vi "Double_Solenoid_Sample.vi"() -> ()   [LabVIEW 2020]
uses:
  <vilib>/Rock Robotics/WPI/Solenoid/WPI_SolenoidChannel.ctl
  <vilib>/Rock Robotics/WPI/Solenoid/WPI_SolenoidValue.ctl
  <vilib>/Rock Robotics/WPI/ThirdParty/JAS_Junk/TrajLib/Timer_New.vi
  <vilib>/Rock Robotics/WPI/Utilities/WPI_GetSetVariantRefNum.vi
  <vilib>/Rock Robotics/WPI/Solenoid/WPI_SolenoidOpenDouble.vi
  <vilib>/Utility/semaphor.llb/Obtain Semaphore Reference.vi
  <vilib>/Rock Robotics/WPI/ThirdParty/JAS_Junk/TrajLib/Timer_Reset.vi
  <vilib>/Rock Robotics/WPI/ThirdParty/JAS_Junk/TrajLib/Timer_Start.vi
  <vilib>/Rock Robotics/WPI/ThirdParty/JAS_Junk/TrajLib/Timer_HasPeriodPassedOnce.vi
  <vilib>/Rock Robotics/WPI/Solenoid/WPI_SolenoidSetEnum.vi
  <vilib>/Rock Robotics/WPI/Solenoid/WPI_SolenoidGetEnum.vi
  <vilib>/Rock Robotics/WPI/ThirdParty/JAS_Junk/TrajLib/Trajectory_Library.lvlib
panel:
  in  "OneShot Time":dbl=0.33 format="%#_13g"
  out "Desired Cmd":T1
  in  "Intake Dmd":bool
  out "Solenoid Value":T1
  in  "Reverse Solenoid Channel":T2=enum."Solenoid 1"
  in  "Forward Solenoid Channel":T2
  in  "Pneumatics Device (def)":u8
  out "Analog  Sensors":cluster{"Analog 0 (V)":dbl, "Analog 1 (V)":dbl}
  out "Pressure Sensors":T3
  out "Compressor Running":bool
  out "Enabled":bool
  out "Solenoid Cmd Chart":cluster{dbl, "mean":dbl}(graph)
  # "Double Solenoid Example"
  # "Set these values before\nexecuting program"
  # "These values can be\nchanged while the \nprogram is running"
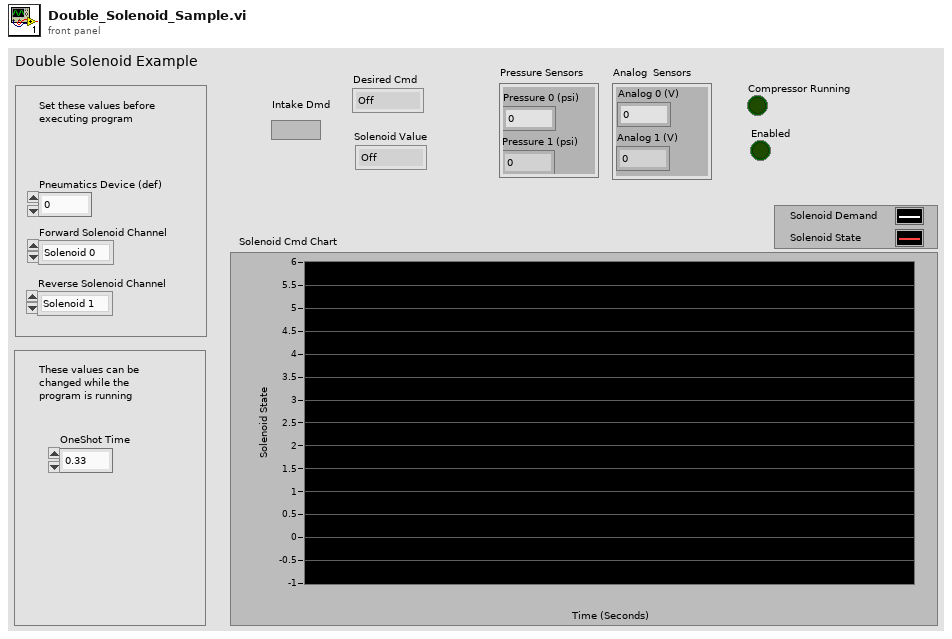
[diagram p1: front panel]
types:
  T1 = typedef "WPI_SolenoidValue.ctl" = enum16{"Off", "On", "Forward", "Reverse"}
  T2 = typedef "WPI_SolenoidChannel.ctl" = enum8{"Solenoid 0", "Solenoid 1", "Solenoid 2", "Solenoid 3", "Solenoid 4", "Solenoid 5", "Solenoid 6", "Solenoid 7", "Solenoid 8", "Solenoid 9", "Solenoid 10", "Solenoid 11", "Solenoid 12", "Solenoid 13", "Solenoid 14", "Solenoid 15", "Invalid"}
  T3 = cluster{"Pressure 0 (psi)":dbl, "Pressure 1 (psi)":dbl}
  T4 = typedef "WPI_CompressorDevRef.ctl" = cluster{"DevStatus":errorcluster, "Pneumatics Control Module":u8}
  T5 = typedef "WPI_SolenoidDevRef.ctl" = cluster{"DevStatus":errorcluster, "Pneumatics Control Module":u8, "Forward Solenoid Channel":T2, "Reverse Solenoid Channel":T2}
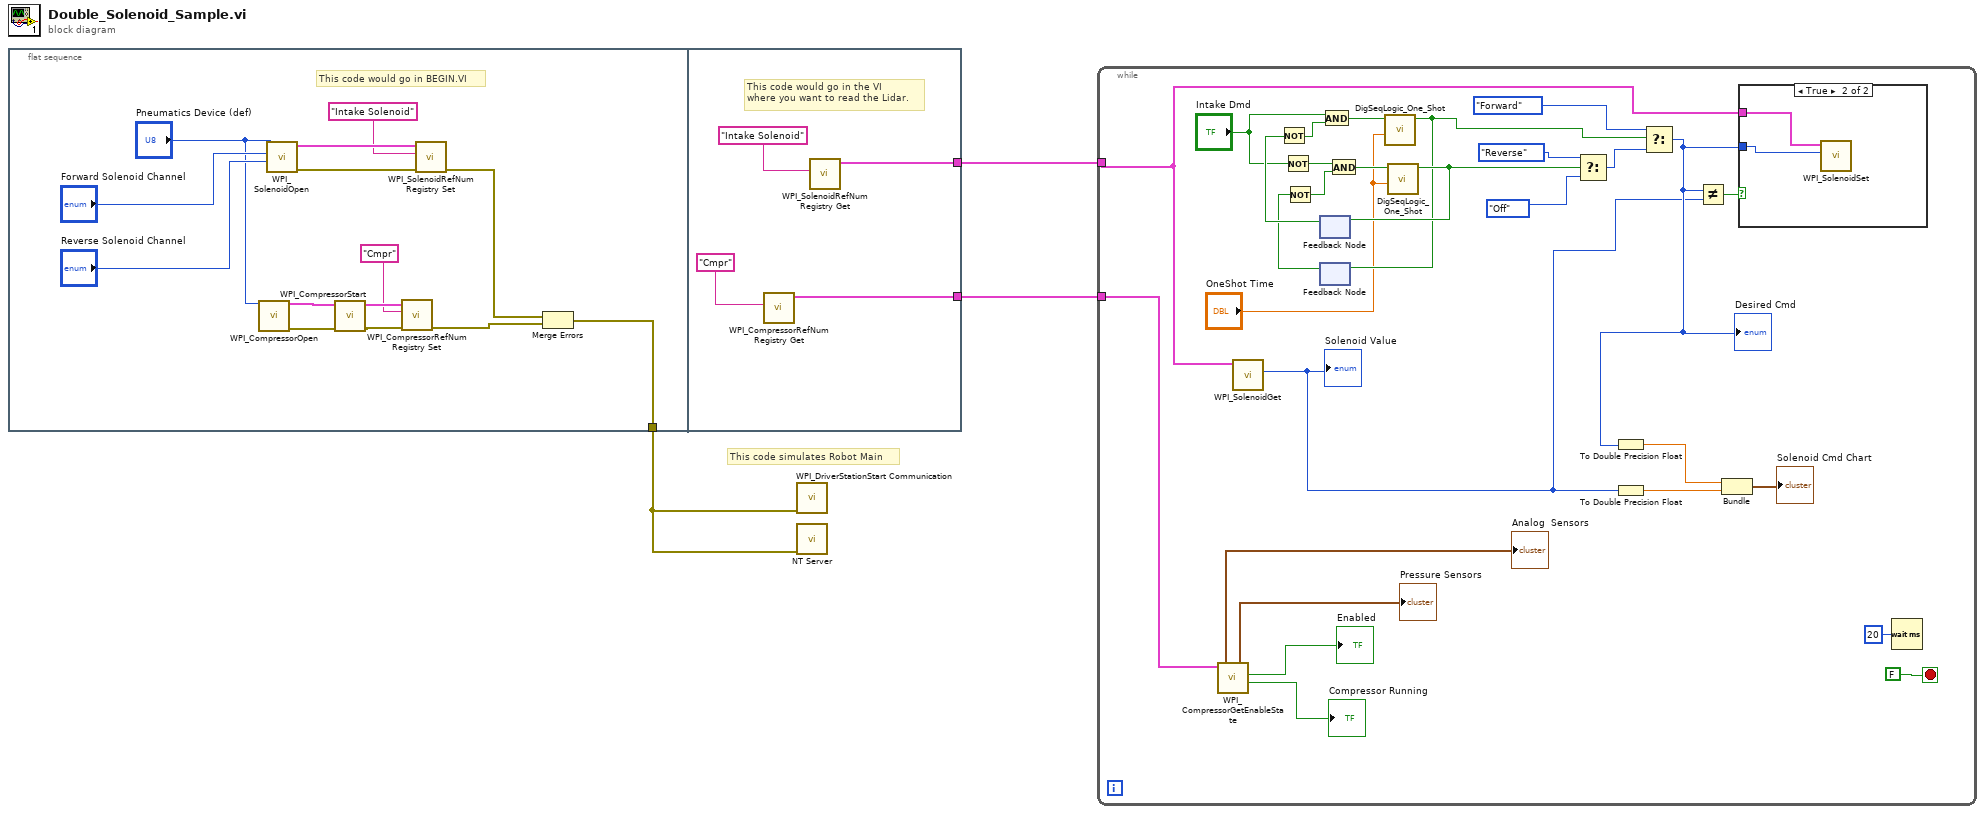
[diagram p0: block diagram]
diagram:
  # "This code simulates Robot Main"
  n1 = flat-sequence {
    tunnel: [w8] -> w3
    tunnel: [w20] -> w2
    tunnel: [w18] -> w1
    frame #0 {
      # "This code would go in BEGIN.VI"
      n2 = call <vilib>:"WPI_CompressorOpen.vi"("Pneumatics device (def)"="Pneumatics Device (def)") -> ("CompressorDevRef"=w16:T4, "error out"=w17:errorcluster)  [unwired: 13 in]
      n3 = call-poly <vilib>:"WPI_SolenoidOpen.vi"("Reverse Solenoid Channel"="Reverse Solenoid Channel", "Forward Solenoid Channel"="Forward Solenoid Channel", "Pneumatics Device (def)"="Pneumatics Device (def)") -> ("error out"=w11:errorcluster, "SolenoidDevRef"=w12:T5)  [unwired: 7 in]
      n4 = call <vilib>:"WPI_CompressorStart.vi"("error in (no error)"=w17, "CompressorDevRef"=w16) -> ("error out"=w13:errorcluster, "CompressorDevRef"=w15:T4)  [unwired: 8 in]
      n5 = call <vilib>:"WPI_CompressorRefNum Registry Set.vi"("error in (no error)"=w13, "refnum name"="Cmpr", "CompressorDevRef"=w15) -> ("error out"=w10:errorcluster)  [unwired: 7 in, 1 out]
      n6 = call <vilib>:"WPI_SolenoidRefNum Registry Set.vi"("error in (no error)"=w11, "refnum name"="Intake Solenoid", "SolenoidDevRef"=w12) -> ("error out"=w9:errorcluster)  [unwired: 7 in, 1 out]
      n7 = Merge Errors(w9, w10) -> (w8:errorcluster)
    }
    frame #1 {
      # "This code would go in the VI\nwhere you want to read the Lidar."
      n8 = call <vilib>:"WPI_CompressorRefNum Registry Get.vi"("refnum name"="Cmpr") -> ("CompressorDevRef"=w20:T4)  [unwired: 9 in, 1 out]
      n9 = call <vilib>:"WPI_SolenoidRefNum Registry Get.vi"("refnum name"="Intake Solenoid") -> ("SolenoidDevRef"=w18:T5)  [unwired: 9 in, 1 out]
    }
  }
  n10 = call <vilib>:"WPI_DriverStationStart Communication.vi"("error in (no error)"=w3) -> ()  [unwired: 11 in]
  n11 = call <vilib>:"NT Server.vi"("error in (no error)"=w3) -> ()  [unwired: 11 in]
  n12 = while {
    tunnel: w2 -> [w48]
    tunnel: w1 -> [w43]
    stop <- FALSE stop-if-true
    n13 = call <vilib>:"WPI_CompressorGetEnableState.vi"("CompressorDevRef"=w48) -> ("Compressor Running"=→"Compressor Running":bool, "Enabled"=→"Enabled":bool, "Pressure Sensors"=→"Pressure Sensors":T3, "Analog  Sensors"=→"Analog  Sensors":cluster{"Analog 0 (V)":dbl, "Analog 1 (V)":dbl})  [unwired: 4 in, 3 out]
    n14 = call-poly <vilib>:"WPI_SolenoidGet.vi"("SolenoidDevRef"=w43) -> ("Value"=w22:T1)  [unwired: 8 in, 2 out]
    "Solenoid Value" <- w22
    n15 = Not(x="Intake Dmd") -> (.not. x?=w31:bool)
    n16 = feedback #1() -> (w33:bool)  [unwired: 1 in]
    n17 = Not(x=w33) -> (.not. x?=w35:bool)
    n18 = feedback #2() -> (w28:bool)  [unwired: 1 in]
    n19 = Not(x=w28) -> (.not. x?=w30:bool)
    n20 = And(x="Intake Dmd", y=w35) -> (x .and. y?=w36:bool)
    n21 = And(x=w31, y=w30) -> (x .and. y?=w37:bool)
    n22 = call <vilib>:"DigSeqLogic_One_Shot.vi"("OneShot"="OneShot Time", "Input"=w36) -> ("Output"=w29:bool)  [unwired: 8 in, 1 out]
    n23 = feedback-in #2(w29) -> ()
    n24 = call <vilib>:"DigSeqLogic_One_Shot.vi"("OneShot"="OneShot Time", "Input"=w37) -> ("Output"=w34:bool)  [unwired: 8 in, 1 out]
    n25 = feedback-in #1(w34) -> ()
    n26 = Select(t=WPI_SolenoidValue."Reverse" ("Value"), s=w34, f=WPI_SolenoidValue."Off" ("Value")) -> (s? t:f=w40:T1)
    n27 = To Double Precision Float(number=w22) -> (double precision float=w23:dbl)
    n28 = Select(t=WPI_SolenoidValue."Forward" ("Value"), s=w29, f=w40) -> (s? t:f=w24:T1)
    "Desired Cmd" <- w24
    n29 = To Double Precision Float(number=w24) -> (double precision float=w25:dbl)
    n30 = Not Equal?(x=w24, y=w22) -> (x != y?=w41:bool)
    n31 = Bundle(w25, w23) -> (→"Solenoid Cmd Chart":cluster{dbl, dbl})  [unwired: 1 in]
    n32 = case shown="True" w41 {
      tunnel: w43 -> [_ w52]
      tunnel: w24 -> [_ w51]
      frame False {
      }
      frame True {
        n33 = call-poly <vilib>:"WPI_SolenoidSet.vi"("Value"=w51, "SolenoidDevRef"=w52) -> ()  [unwired: 8 in, 2 out]
      }
    }
    n34 = Wait (ms)(milliseconds to wait=u32 20) -> ()  [unwired: 1 out]
  }
